vi "实验内容_实验选择界面.vi"() -> ()   [LabVIEW 2014]
panel:
  in  "实验选择":T1=1 items=["请选择实验...", "X射线特征谱测量及Ｘ射线吸收", "α粒子能量损失", "β射线吸收", "γ能量测量实验", "放射性半衰期"]
  in  "退出":bool
  in  "确定":bool
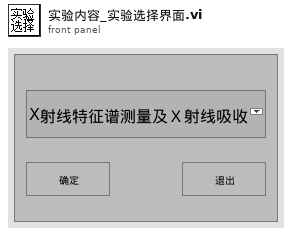
[diagram p1: front panel]
types:
  T1 = typedef "实验内容_实验选择界面.ctl" = u16
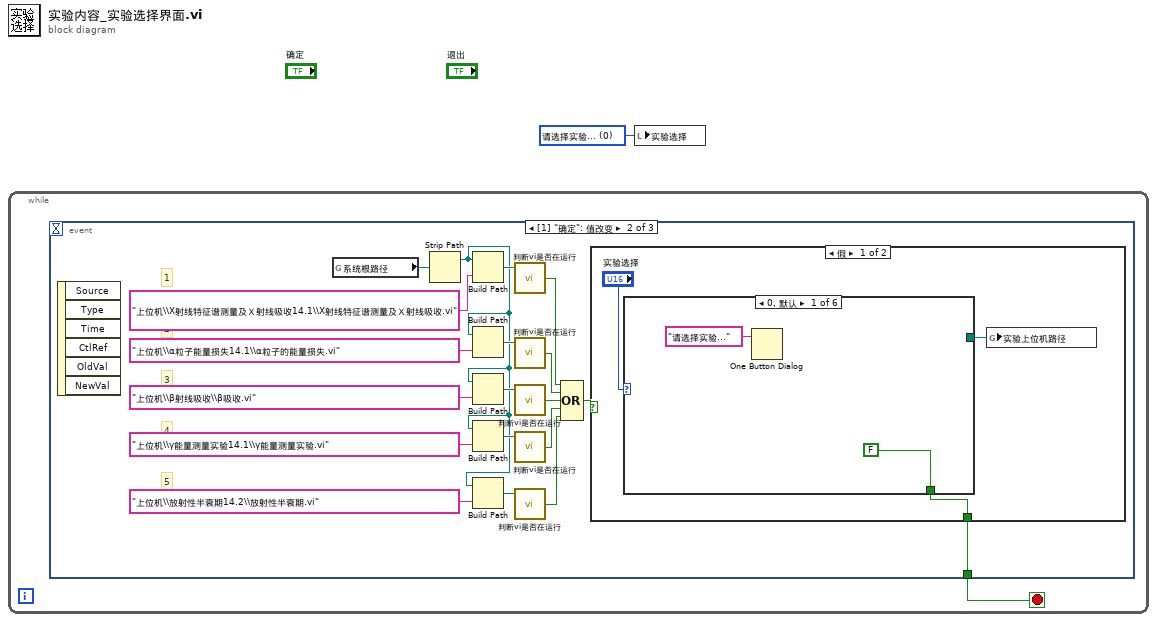
[diagram p0: block diagram]
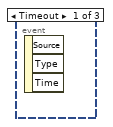
[diagram p2: hidden frame]
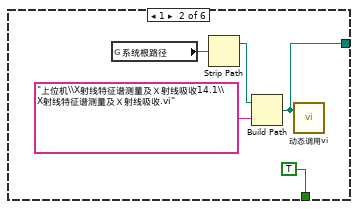
[diagram p3: hidden frame]
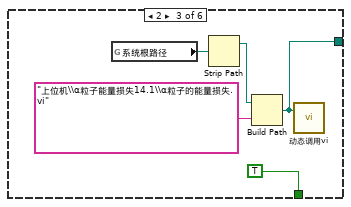
[diagram p4: hidden frame]
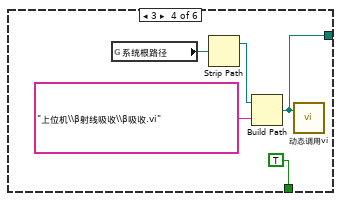
[diagram p5: hidden frame]
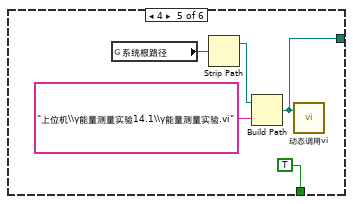
[diagram p6: hidden frame]
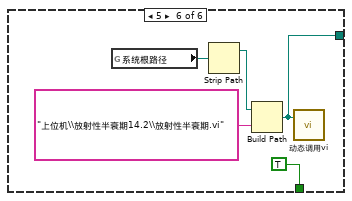
[diagram p7: hidden frame]
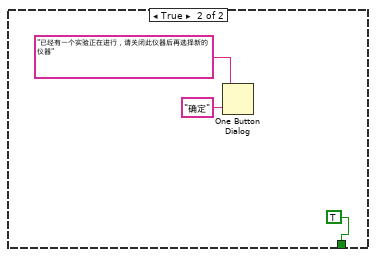
[diagram p8: hidden frame]
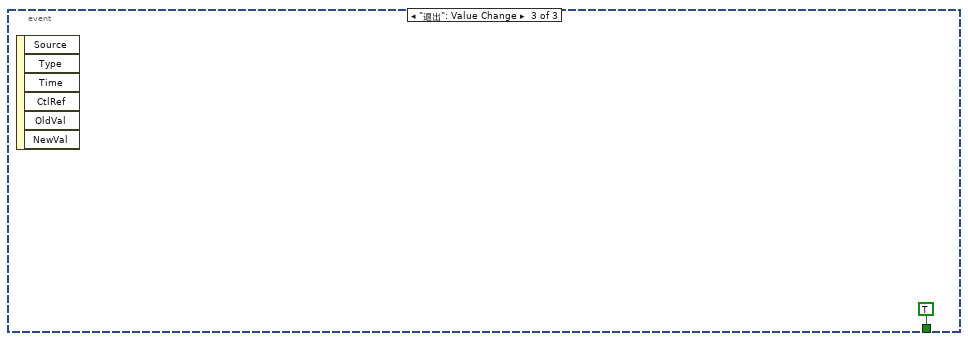
[diagram p9: hidden frame]
diagram:
  w1 = T1 0 items=["请选择实验...", "X射线特征谱测量及Ｘ射线吸收", "α粒子能量损失", "β射线吸收", "γ能量测量实验", "放射性半衰期"] ("仪器选择")
  n1 = while {
    stop <- w2 stop-if-true
    n2 = event shown="[1] \"确定\": 值改变" {
      selector: _ -> [_ _ _]
      dyn-events: _ -> [_ _ _]
      timeout: _ -> [_ _ _]
      tunnel: [_ w3 TRUE] -> w2
      event Timeout {
        n3 = event-data() -> ()  [unwired: 1 in, 3 out]
      }
      event "确定": Value Change {
        # "5"
        # "4"
        # "3"
        # "2"
        # "1"
        n4 = event-data() -> ()  [unwired: 1 in, 6 out]
        n5 = global read "系统全局变量.vi" "系统根路径"() -> (w21:path)
        n6 = Strip Path(path=w21) -> (stripped path=w5:path)  [unwired: 1 out]
        n7 = Build Path(base path=w5, name or relative path="上位机\\X射线特征谱测量及Ｘ射线吸收14.1\\X射线特征谱测量及Ｘ射线吸收.vi" ("名称或相对路径")) -> (appended path=w19:path)
        n8 = Build Path(base path=w5, name or relative path="上位机\\α粒子能量损失14.1\\α粒子的能量损失.vi" ("名称或相对路径")) -> (appended path=w18:path)
        n9 = Build Path(base path=w5, name or relative path="上位机\\β射线吸收\\β吸收.vi" ("名称或相对路径")) -> (appended path=w15:path)
        n10 = Build Path(base path=w5, name or relative path="上位机\\γ能量测量实验14.1\\γ能量测量实验.vi" ("名称或相对路径")) -> (appended path=w14:path)
        n11 = Build Path(base path=w5, name or relative path="上位机\\放射性半衰期14.2\\放射性半衰期.vi" ("名称或相对路径")) -> (appended path=w6:path)
        n12 = call "判断vi是否在运行.vi"("VI路径"=w19) -> ("vi正在运行?"=w12:bool)  [unwired: 2 in, 2 out]
        n13 = call "判断vi是否在运行.vi"("VI路径"=w18) -> ("vi正在运行?"=w11:bool)  [unwired: 2 in, 2 out]
        n14 = call "判断vi是否在运行.vi"("VI路径"=w15) -> ("vi正在运行?"=w10:bool)  [unwired: 2 in, 2 out]
        n15 = call "判断vi是否在运行.vi"("VI路径"=w14) -> ("vi正在运行?"=w9:bool)  [unwired: 2 in, 2 out]
        n16 = call "判断vi是否在运行.vi"("VI路径"=w6) -> ("vi正在运行?"=w4:bool)  [unwired: 2 in, 2 out]
        n17 = Compound Arithmetic op=OR(w12, w11, w10, w9, w4) -> (w8:bool)
        n18 = case shown="假" w8 {
          tunnel: [w23 TRUE] -> w3
          frame False {
            n19 = case shown="0, 默认" "实验选择" {
              tunnel: [FALSE TRUE TRUE TRUE TRUE TRUE] -> w23
              tunnel: [_ w27 w32 w37 w42 w47] -> w22
              frame 0, Default {
                n20 = One Button Dialog(message="请选择实验..." ("消息")) -> ()  [unwired: 1 in, 1 out]
              }
              frame 1 {
                n21 = global read "系统全局变量.vi" "系统根路径"() -> (w29:path)
                n22 = Strip Path(path=w29) -> (stripped path=w30:path)  [unwired: 1 out]
                n23 = Build Path(base path=w30, name or relative path="上位机\\X射线特征谱测量及Ｘ射线吸收14.1\\X射线特征谱测量及Ｘ射线吸收.vi" ("名称或相对路径")) -> (appended path=w27:path)
                n24 = call "动态调用vi.vi"("VI路径"=w27) -> ()  [unwired: 1 in, 1 out]
              }
              frame 2 {
                n25 = global read "系统全局变量.vi" "系统根路径"() -> (w34:path)
                n26 = Strip Path(path=w34) -> (stripped path=w35:path)  [unwired: 1 out]
                n27 = Build Path(base path=w35, name or relative path="上位机\\α粒子能量损失14.1\\α粒子的能量损失.vi" ("名称或相对路径")) -> (appended path=w32:path)
                n28 = call "动态调用vi.vi"("VI路径"=w32) -> ()  [unwired: 1 in, 1 out]
              }
              frame 3 {
                n29 = global read "系统全局变量.vi" "系统根路径"() -> (w39:path)
                n30 = Strip Path(path=w39) -> (stripped path=w40:path)  [unwired: 1 out]
                n31 = Build Path(base path=w40, name or relative path="上位机\\β射线吸收\\β吸收.vi" ("名称或相对路径")) -> (appended path=w37:path)
                n32 = call "动态调用vi.vi"("VI路径"=w37) -> ()  [unwired: 1 in, 1 out]
              }
              frame 4 {
                n33 = global read "系统全局变量.vi" "系统根路径"() -> (w44:path)
                n34 = Strip Path(path=w44) -> (stripped path=w45:path)  [unwired: 1 out]
                n35 = Build Path(base path=w45, name or relative path="上位机\\γ能量测量实验14.1\\γ能量测量实验.vi" ("名称或相对路径")) -> (appended path=w42:path)
                n36 = call "动态调用vi.vi"("VI路径"=w42) -> ()  [unwired: 1 in, 1 out]
              }
              frame 5 {
                n37 = global read "系统全局变量.vi" "系统根路径"() -> (w49:path)
                n38 = Strip Path(path=w49) -> (stripped path=w50:path)  [unwired: 1 out]
                n39 = Build Path(base path=w50, name or relative path="上位机\\放射性半衰期14.2\\放射性半衰期.vi" ("名称或相对路径")) -> (appended path=w47:path)
                n40 = call "动态调用vi.vi"("VI路径"=w47) -> ()  [unwired: 1 in, 1 out]
              }
            }
            n41 = global write "系统全局变量.vi" "实验上位机路径"(w22) -> ()
          }
          frame True {
            n42 = One Button Dialog(message="已经有一个实验正在进行，请关闭此仪器后再选择新的仪器" ("消息"), button name ("OK")="确定" ("按钮名称（“确定”）")) -> ()  [unwired: 1 out]
          }
        }
      }
      event "退出": Value Change {
        n43 = event-data() -> ()  [unwired: 1 in, 6 out]
      }
    }
  }
  n44 = local write "实验选择"(w1) -> ()
